vi "API - DIO - Enable Digital Output.vi"(8 "error in":errorcluster, 10 "Channel Number":i32, 11 "DAQiFi Device Properties In":T1) -> (0 "error out":errorcluster, 3 "DAQiFi Device Properties Out":T1)   [LabVIEW 2021]
doc: "Enables the DIO port, and sets the digital line to be an output."
uses:
  TypeDefs/TypeDef - Cluster of DAQiFi Device Properties.ctl
  TypeDefs/Enum - Connection Type.ctl
  TCP - Write and Read a Synchronous Message.vi
  USB - Write and Read a Synchronous Message.vi
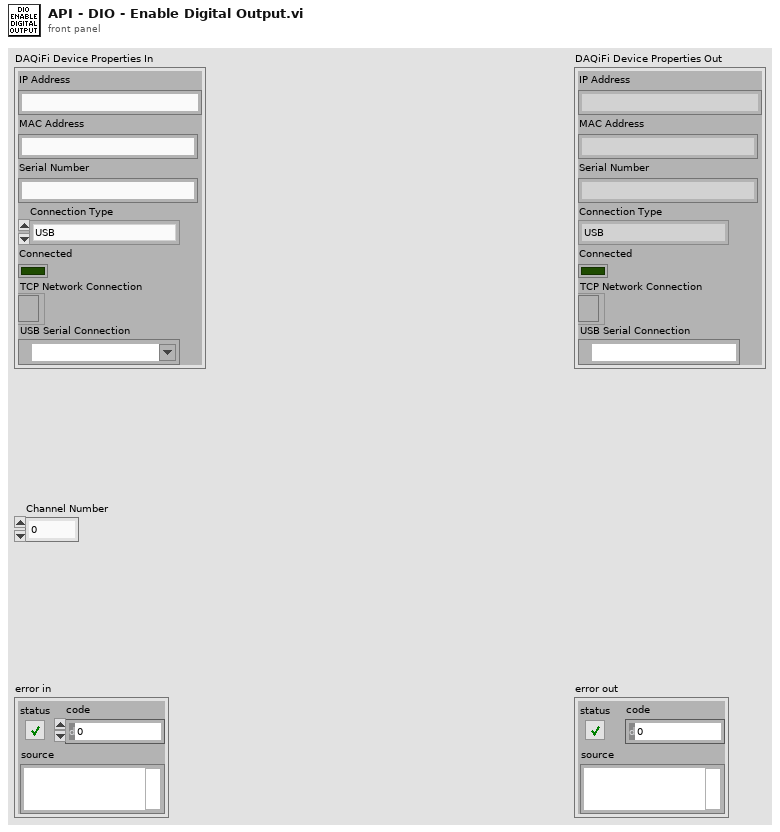
[diagram p1: front panel]
types:
  T1 = typedef "TypeDef - Cluster of DAQiFi Device Properties.ctl" = cluster{"IP Address":string, "MAC Address":string, "Serial Number":string, "Connection Type":T2, "Connected":bool, "TCP Network Connection":refnum<k5>, "USB Serial Connection":refnum<visa-resource-name>}
  T2 = typedef "Enum - Connection Type.ctl" = enum16{"USB", "TCP"}
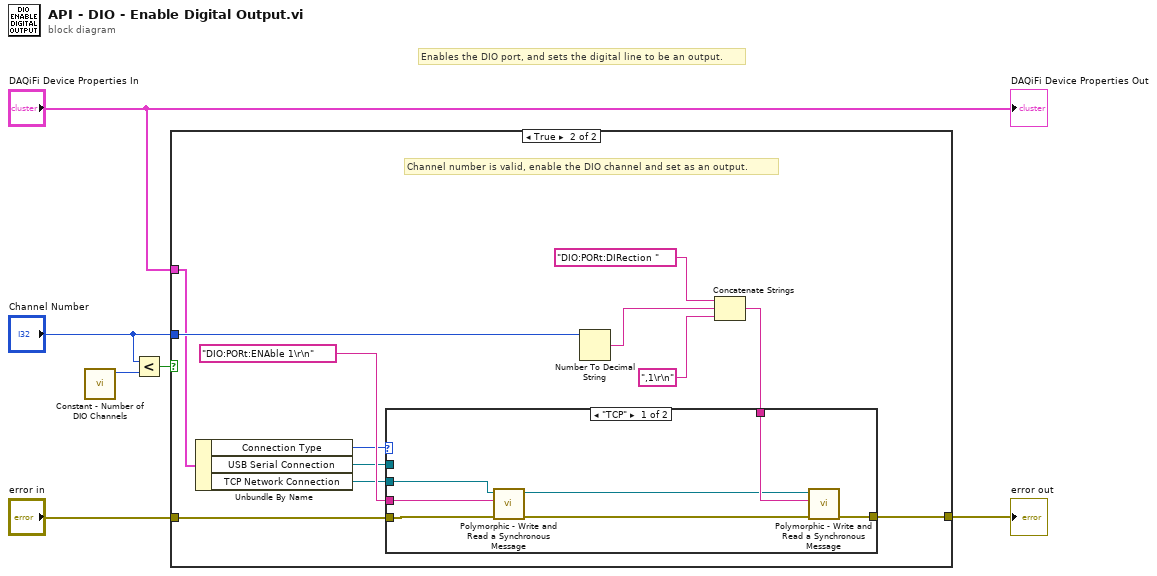
[diagram p0: block diagram]
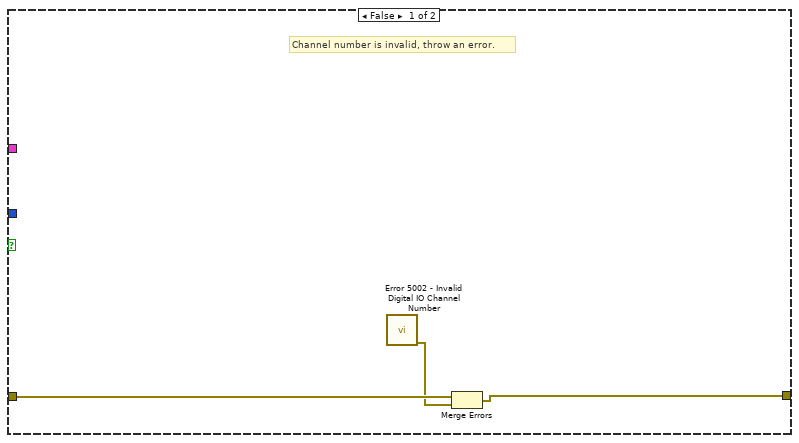
[diagram p2: hidden frame]
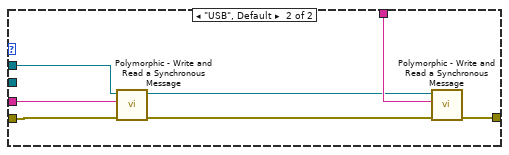
[diagram p3: hidden frame]
diagram:
  # "Enables the DIO port, and sets the digital line to be an output."
  n1 = call "Constant - Number of DIO Channels.vi"() -> ("Maximum Channel"=w3:i32)  [unwired: 11 in]
  n2 = Less?(x="Channel Number", y=w3) -> (x < y?=w2:bool)
  n3 = case shown="True" w2 {
    tunnel: "error in" -> [w9 w21]
    tunnel: [w7 w19] -> w5
    tunnel: "Channel Number" -> [_ w14]
    tunnel: "DAQiFi Device Properties In" -> [_ w13]
    frame False {
      # "Channel number is invalid, throw an error."
      n4 = call "Error 5002 - Invalid Digital IO Channel Number.vi"() -> ("error out"=w8:errorcluster)  [unwired: 11 in]
      n5 = Merge Errors(w9, w8) -> (w7:errorcluster)
    }
    frame True {
      # "Channel number is valid, enable the DIO channel and set as an output."
      n6 = Unbundle By Name(w13) -> ("Connection Type"=w12:T2, "USB Serial Connection"=w10:refnum<visa-resource-name>, "TCP Network Connection"=w11:refnum<k5>)
      n7 = Number To Decimal String(number=w14) -> (decimal integer string=w16:string)  [unwired: 1 in]
      n8 = Concatenate Strings("DIO:PORt:DIRection " ("Message to Send"), w16, ",1\r\n" ("string")) -> (w17:string)
      n9 = case shown="\"TCP\"" w12 {
        tunnel: w21 -> [w28 w35]
        tunnel: "DIO:PORt:ENAble 1\r\n" ("Message to Send") -> [w24 w31]
        tunnel: [w26 w33] -> w19
        tunnel: w17 -> [w25 w32]
        tunnel: w11 -> [w23 _]
        tunnel: w10 -> [_ w29]
        frame "TCP" {
          n10 = call-poly "Polymorphic - Write and Read a Synchronous Message.vi"("error in"=w28, "Message to Send"=w24, "TCP Network Connection in"=w23) -> ("error out"=w27:errorcluster, "TCP Network Connection out"=w22:refnum<k5>)  [unwired: 6 in, 1 out]
          n11 = call-poly "Polymorphic - Write and Read a Synchronous Message.vi"("error in"=w27, "Message to Send"=w25, "TCP Network Connection in"=w22) -> ("error out"=w26:errorcluster)  [unwired: 6 in, 2 out]
        }
        frame "USB", Default {
          n12 = call-poly "Polymorphic - Write and Read a Synchronous Message.vi"("error in"=w35, "Message to Send"=w31, "VISA resource name in"=w29) -> ("error out"=w34:errorcluster, "VISA resource name out"=w30:refnum<visa-resource-name>)  [unwired: 6 in, 1 out]
          n13 = call-poly "Polymorphic - Write and Read a Synchronous Message.vi"("error in"=w34, "Message to Send"=w32, "VISA resource name in"=w30) -> ("error out"=w33:errorcluster)  [unwired: 6 in, 2 out]
        }
      }
    }
  }
  "error out" <- w5
  "DAQiFi Device Properties Out" <- "DAQiFi Device Properties In"
